vi "_Yt09_FAILJUMP.vi"(11 "YTESTER测试数据":T1) -> (3 "YTESTER结论":T2)   [LabVIEW 2017]
doc: "VIClassID=YT_SSTEPFLAG_FAILJUMP\nVIDescription=如果前面失败的话可以跳转某一位置进行重测，测试表也会更新掉。注意，也可以往后跳"
uses:
  YtCommon.lvlibp/yt`Step StepBaseInput.ctl
  YtCommon.lvlibp/yt`Step StepResult.ctl
  YtCommon.lvlibp/yt`Step TestData.ctl
  YtCommon.lvlibp/yt`Step System Queue.ctl
  Step`s VIs/YYLLGeneric/variable_W.ctl
  YtCommon.lvlibp/yt`Data-Ytester Type Data.ctl
  95978aca-67fc-4424-a0ff-2c2ef8b219f8.vi
  <vilib>/Utility/error.llb/Clear Errors.vi
  YtCommon.lvlibp/yt`varSystemlib IO Read Variable.vi
  YtCommon.lvlibp
panel:
  in  "YTESTER开放参数":T4={"YTESTER_BaseInput"={"isTest"=FALSE, "isSkip"=FALSE, "StepName"="重测跳转器", "OnPass"=enum."Next", "OnFail"=enum."Next", "ReTestNumber"=0.0}, "重测跳转器名（空使用StepName）"="", "判断起始行(from1)"=1, "重测最大次数"=1, "跳转目标行(from1)"=1}
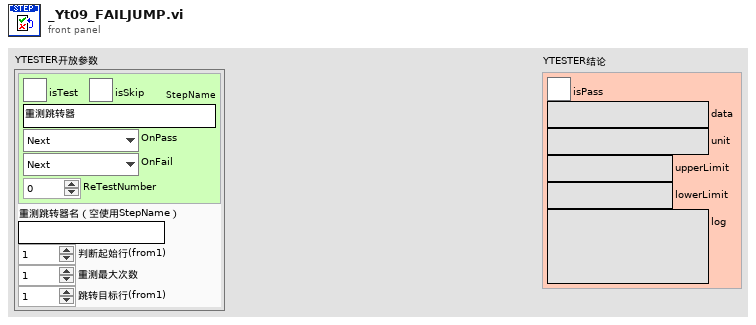
[diagram p1: front panel]
types:
  T1 = typedef "YtCommon.lvlibp/yt`Step TestData.ctl" = cluster{"Socket(From1)":i32, "SN":refnum<notifier>, "StopFlagRef":refnum<notifier>, "YT System Queue":refnum<queue>}
  T2 = typedef "YtCommon.lvlibp/yt`Step StepResult.ctl" = cluster{"isPass":bool, "data":string, "unit":string, "upperLimit":string, "lowerLimit":string, "log":string}
  T3 = typedef "YtCommon.lvlibp/yt`Step StepBaseInput.ctl" = cluster{"isTest":bool, "isSkip":bool, "StepName":string, "OnPass":enum16{"Next", "ToOVER", "Terminate"}, "OnFail":enum16{"Next", "ToOVER", "Terminate"}, "ReTestNumber":dbl}
  T4 = cluster{"YTESTER_BaseInput":T3, "重测跳转器名（空使用StepName）":string, "判断起始行(from1)":u32, "重测最大次数":u32, "跳转目标行(from1)":u32}
  T5 = typedef "variable_W.ctl" = cluster{"YT_TYPE":T6, "TypeData":string[], "Tips":string}
  T6 = typedef "YtCommon.lvlibp/yt`Data-Ytester Type Data.ctl" = enum16{"NULL", "NUM", "BOOL", "TXT", "ENUM", "TIME", "PATH", "VISA", "COMBO", "ColorBox", "RadioBtn", "Array_NUM", "Array_BOOL", "Array_TXT", "Array_ENUM", "Array_PATH", "Array_COMBO"}
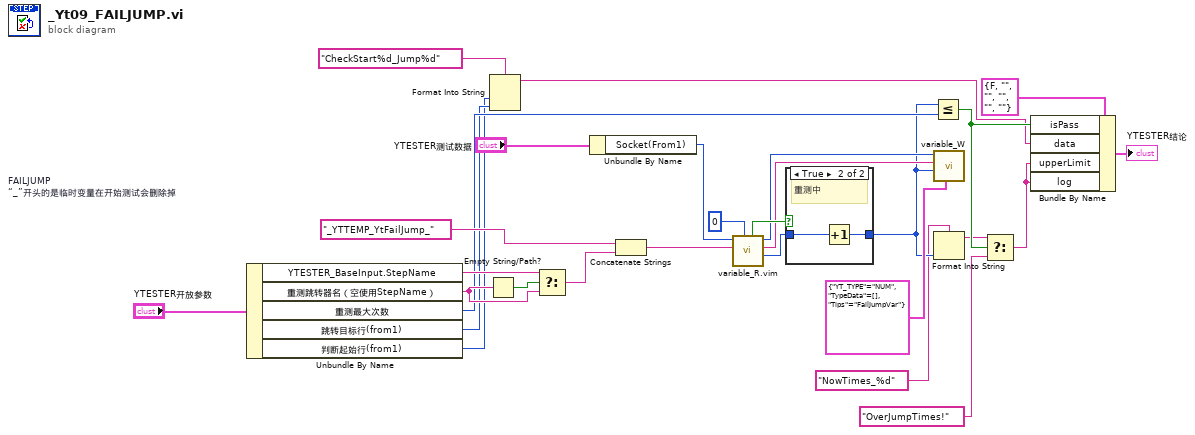
[diagram p0: block diagram]
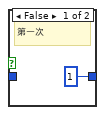
[diagram p2: hidden frame]
diagram:
  w19 = "_YTTEMP_YtFailJump_"  # FAILJUMP “_”开头的是临时变量在开始测试会删除掉
  n1 = Unbundle By Name("YTESTER开放参数") -> ("YTESTER_BaseInput.StepName"=w20:string, "重测跳转器名（空使用StepName）"=w21:string, "重测最大次数"=w11:u32, "跳转目标行(from1)"=w8:u32, "判断起始行(from1)"=w7:u32)
  n2 = Empty String/Path?(string/path=w21) -> (empty?=w26:bool)
  n3 = Format Into String(format string="CheckStart%d_Jump%d", w7, w8) -> (resulting string=w5:string)  [unwired: 2 in, 1 out]
  n4 = Select(t=w20, s=w26, f=w21) -> (s? t:f=w25:string)
  n5 = Unbundle By Name("YTESTER测试数据") -> ("Socket(From1)"=w17:i32)
  n6 = Concatenate Strings(w19, w25) -> (w24:string)
  n7 = call "variable_R.vim"("type"=u32 0 ("函数池名称"), "待获取变量名称"=w24, "函数池名称"=w17) -> ("value"=w13:u32, "待获取变量名out"=w14:string, "函数池名称out"=w15:i32, "found?"=w16:bool)  [unwired: 4 in, 1 out]
  n8 = case shown="True" w16 {
    tunnel: w13 -> [_ w31]
    tunnel: [u32 1 w30] -> w3
    frame False {
      # "第一次"
    }
    frame True {
      # "重测中"
      n9 = Increment(x=w31) -> (x+1=w30:u32)
    }
  }
  n10 = Less Or Equal?(x=w3, y=w11) -> (x <= y?=w10:bool)
  n11 = call "variable_W.vi"("附加的Information"=T5 {"YT_TYPE"=enum."NUM", "TypeData"=[], "Tips"="FailJumpVar"}, "待写入池的输入控件"=w3, "待写入池变量名称"=w14, "函数池名称 in"=w15) -> ()  [unwired: 5 in, 3 out]
  n12 = Format Into String(format string="NowTimes_%d", w3) -> (resulting string=w2:string)  [unwired: 2 in, 1 out]
  n13 = Select(t=w2, s=w10, f="OverJumpTimes!") -> (s? t:f=w4:string)
  n14 = Bundle By Name(cluster=T2 {"isPass"=FALSE, "data"="", "unit"="", "upperLimit"="", "lowerLimit"="", "log"=""} ("Result"), "isPass"=w10, "data"=w5, "upperLimit"=w4, "log"=w4) -> (→"YTESTER结论":T2)
